vi "Check_Key_Name.vi"(11 "String":string) -> (1 "multi?":bool, 2 "IDs":u32[](array[numeric]) format="%x", 3 "ID":u32 format="%x")   [LabVIEW 2023, in "LP_CRC.lvlib"]
uses:
  LP_CRC.lvlib
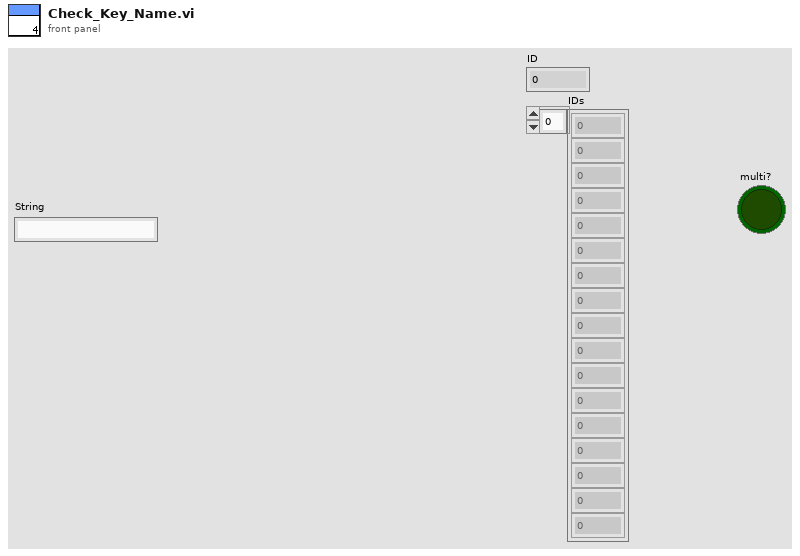
[diagram p1: front panel]
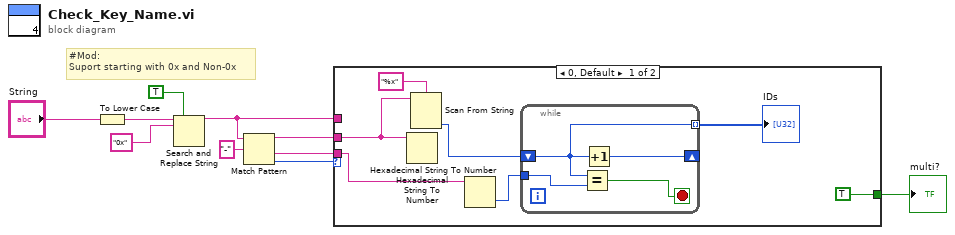
[diagram p0: block diagram]
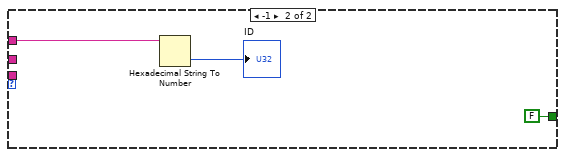
[diagram p2: hidden frame]
diagram:
  # "#Mod:\nSuport starting with 0x and Non-0x"
  n1 = To Lower Case(string="String") -> (all lower case string=w4:string)
  n2 = Search and Replace String(replace all?=TRUE ("replace all? (F)"), input string=w4, search string="0x") -> (result string=w2:string)  [unwired: 5 in, 3 out]
  n3 = Match Pattern(string=w2, regular expression="-") -> (before substring=w8:string, after substring=w7:string, offset past match=w9:i32)  [unwired: 1 in, 1 out]
  n4 = case shown="0, Default" w9 {
    tunnel: w8 -> [w13 _]
    tunnel: w7 -> [w17 _]
    tunnel: w2 -> [_ w23]
    tunnel: [TRUE FALSE] -> w6
    frame 0, Default {
      n5 = Hexadecimal String To Number(string=w13) -> ()  [unwired: 2 in, 2 out]
      n6 = Scan From String(format string="%x", input string=w13) -> (output 1=w11:u32)  [unwired: 3 in, 3 out]
      n7 = Hexadecimal String To Number(string=w17) -> (number=w16:u32)  [unwired: 2 in, 1 out]
      n8 = while {
        tunnel: w16 -> [w19]
        shift-right: [w21] -> _
        shift-left: w11 -> [w20]
        tunnel: [w20] -> w14 mode=indexing
        stop <- w18 stop-if-true
        n9 = Equal?(x=w20, y=w19) -> (x = y?=w18:bool)
        n10 = Increment(x=w20) -> (x+1=w21:u32)
      }
      "IDs" <- w14
    }
    frame -1 {
      n11 = Hexadecimal String To Number(string=w23) -> (number=→"ID":u32)  [unwired: 2 in, 1 out]
    }
  }
  "multi?" <- w6
